vi "Helm Pack Heading Msg.vi"(8 "error in (no error)":errorcluster, 11 "Heading Command Control":T1) -> (0 "error out":errorcluster, 3 "Heading Command Msg out":refnum<class "Heading Command Msg.lvclass">)   [LabVIEW 2015, in "RDS Helm Actor.lvlib"]
uses:
  RDS Helm Actor.lvlib
  Libraries/RDS Child Messages/Helm/Heading Command/Heading Command Cntrl.ctl
  Libraries/RDS Child Messages/Helm/Heading Command/Heading Command Msg.lvclass
  Libraries/RDS Framework/RDS Message ID.ctl
  Libraries/RDS Framework/RDS Message Class/RDS Message.lvclass/RDS Message.ctl
  Libraries/RDS Child Messages/Helm/Heading Command/Heading Command Msg.lvclass/Heading Command Msg.ctl
  Libraries/RDS Framework/RDS Message Class/RDS Message.lvclass
  Libraries/RDS Child Messages/RDS Child Messages.lvlib
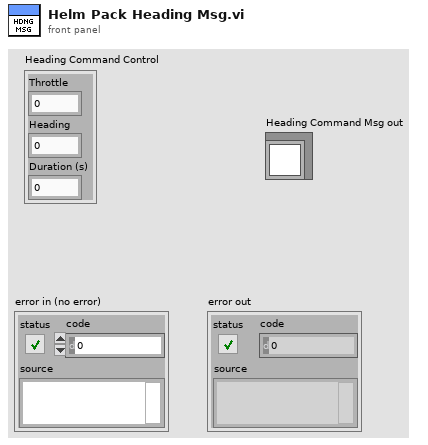
[diagram p1: front panel]
types:
  T1 = typedef "RDS Child Messages.lvlib/Heading Command Cntrl.ctl" = cluster{"Throttle":i16, "Heading":sgl, "Duration (s)":i16}
  T2 = typedef "RDS Child Messages.lvlib/RDS Message ID.ctl" = enum16{"RDS Hello World", "String Message", "AIP_Status", "AIP_Command", "GPS_Data", "MCB_Command", "MCB_Status", "Compass_Data", "Depth_Data", "Battery_Data", "Contoller_State", "Set_Mag_Dev", "BTB_Shutdown", "State_Sample_Request", "State_Sample", "PID_Gains_Set", "Helm_Limiter_Set", "Helm_Heading_Command", "Helm_Steering_Command", "Helm_Status", "Controller_Message", "AIP_Set_Min_Depth", "Mission_Controller_State", "Mission_Upload", "Mission_Set_Op_and_Run", "Mission_Settings_Set"}
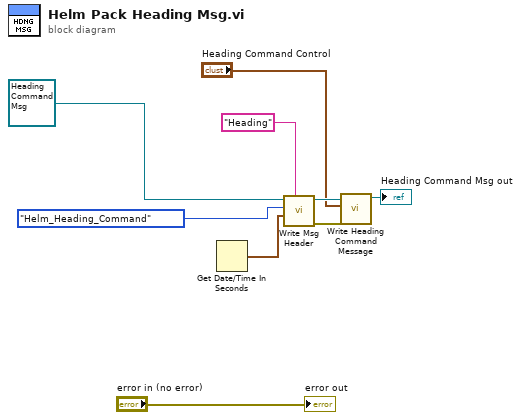
[diagram p0: block diagram]
diagram:
  n1 = Get Date/Time In Seconds() -> (seconds since 1Jan1904=w7:timestamp)
  n2 = call "Write Msg Header.vi"("Sender Name"="Heading", "Time Stamp"=w7, "Msg ID"=RDS_Message_ID."Helm_Heading_Command", "RDS Message in"=refnum<class "Heading Command Msg.lvclass"> refnum ("RDS Child Messages.lvlib:Heading Command Msg.lvclass")) -> ("error out"=w4:errorcluster, "RDS Message out"=w3:refnum<class "Heading Command Msg.lvclass">)  [unwired: 6 in]
  n3 = call "Write Heading Command Message.vi"("error in (no error)"=w4, "Heading Command Control"="Heading Command Control", "Heading Command Msg in"=w3) -> ("Heading Command Msg out"=→"Heading Command Msg out":refnum<class "Heading Command Msg.lvclass">)  [unwired: 7 in, 1 out]
  "error out" <- "error in (no error)"
